vi "Initiate variables.vi"(0 "1D ANN":i32[](array[numeric])) -> (1 "1D ANN":i32[](array[numeric]), 2 "3D W":dbl[][][](array[numeric]) format="%.2f", 3 "3D dW":dbl[][][](array[numeric]) format="%.2f", 4 "N out":dbl[][](array[numeric]) format="%.2f")   [LabVIEW 2010]
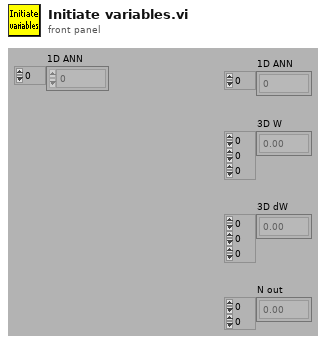
[diagram p1: front panel]
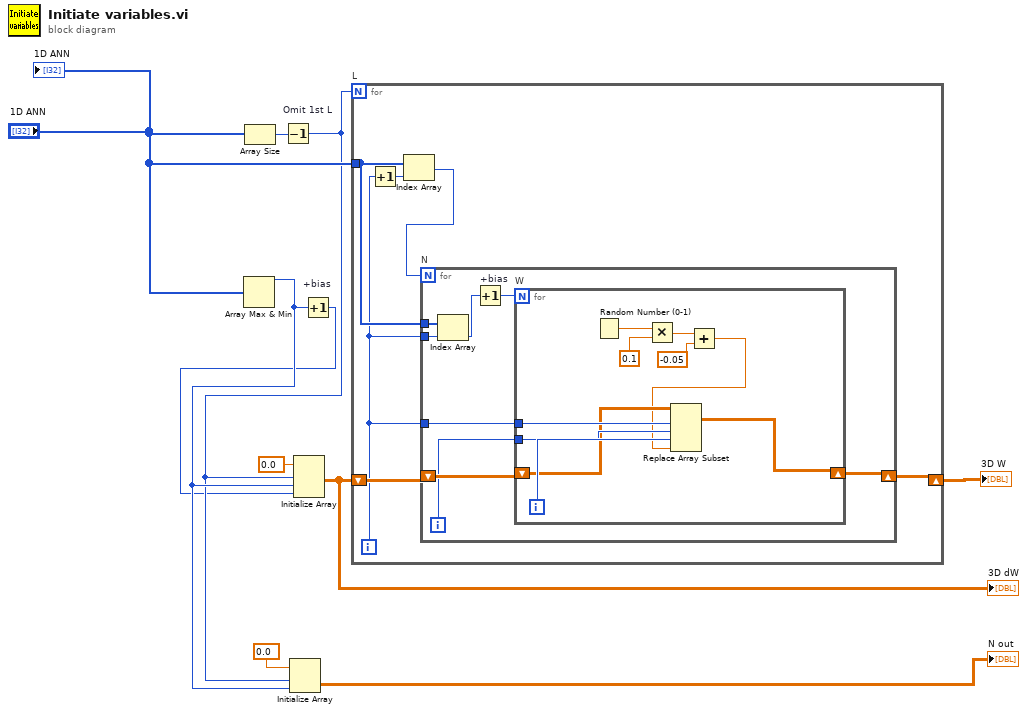
[diagram p0: block diagram]
diagram:
  n1 = Array Max & Min(array="1D ANN") -> (max value=w7:i32)  [unwired: 3 out]
  n2 = Array Size(array="1D ANN") -> (size(s)=w1:i32)
  n3 = Decrement "Omit 1st L"(x=w1) -> (x-1=w6:i32)
  n4 = Initialize Array(0.0 ("Element Data"), w6, w7) -> (→"N out":dbl[][])
  n5 = Increment "+bias"(x=w7) -> (x+1=w4:i32)
  n6 = Initialize Array(0.0 ("Element Data"), w6, w7, w4) -> (w9:dbl[][][])
  "3D dW" <- w9
  n7 = for "L" {
    N: w6 -> [_]
    shift-right: [w15] -> w2
    shift-left: w9 -> [w16]
    tunnel: "1D ANN" -> [w12]
    i -> [w11]
    n8 = Increment(x=w11) -> (x+1=w14:i32)
    n9 = Index Array(array=w12, index=w14) -> (element=w13:i32)
    n10 = for "N" {
      N: w13 -> [_]
      shift-right: [w23] -> w15
      shift-left: w16 -> [w24]
      tunnel: w11 -> [w22]
      tunnel: w12 -> [w20]
      tunnel: w11 -> [w19]
      i -> [w21]
      n11 = Index Array(array=w20, index=w19) -> (element=w18:i32)
      n12 = Increment "+bias"(x=w18) -> (x+1=w17:i32)
      n13 = for "W" {
        N: w17 -> [_]
        shift-right: [w31] -> w23
        shift-left: w24 -> [w30]
        tunnel: w22 -> [w32]
        tunnel: w21 -> [w33]
        i -> [w34]
        n14 = Random Number (0-1)() -> (number: 0 to 1=w29:dbl)
        n15 = Multiply(x=w29, y=0.1) -> (x*y=w27:dbl)
        n16 = Add(x=w27, y=-0.05) -> (x+y=w25:dbl)
        n17 = Replace Array Subset(array=w30, new element=w25, index (dim 0)=w32, index (dim 1)=w33, index (dim 2)=w34) -> (w31:dbl[][][])
      }
    }
  }
  "3D W" <- w2
  "1D ANN" <- "1D ANN"
